vi "Auto 11.vi"(8 "Error In":errorcluster) -> (0 "Error Out":errorcluster)   [LabVIEW 2014]
uses:
  Global Variables/Refnum Names.vi
  <vilib>/Rock Robotics/Network Tables/SD Read Number.vi
  <vilib>/Rock Robotics/Network Tables/SD Read Boolean.vi
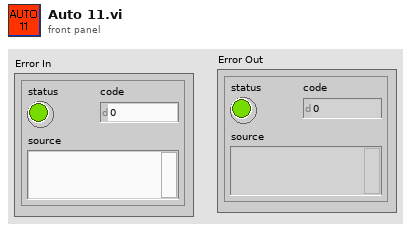
[diagram p1: front panel]
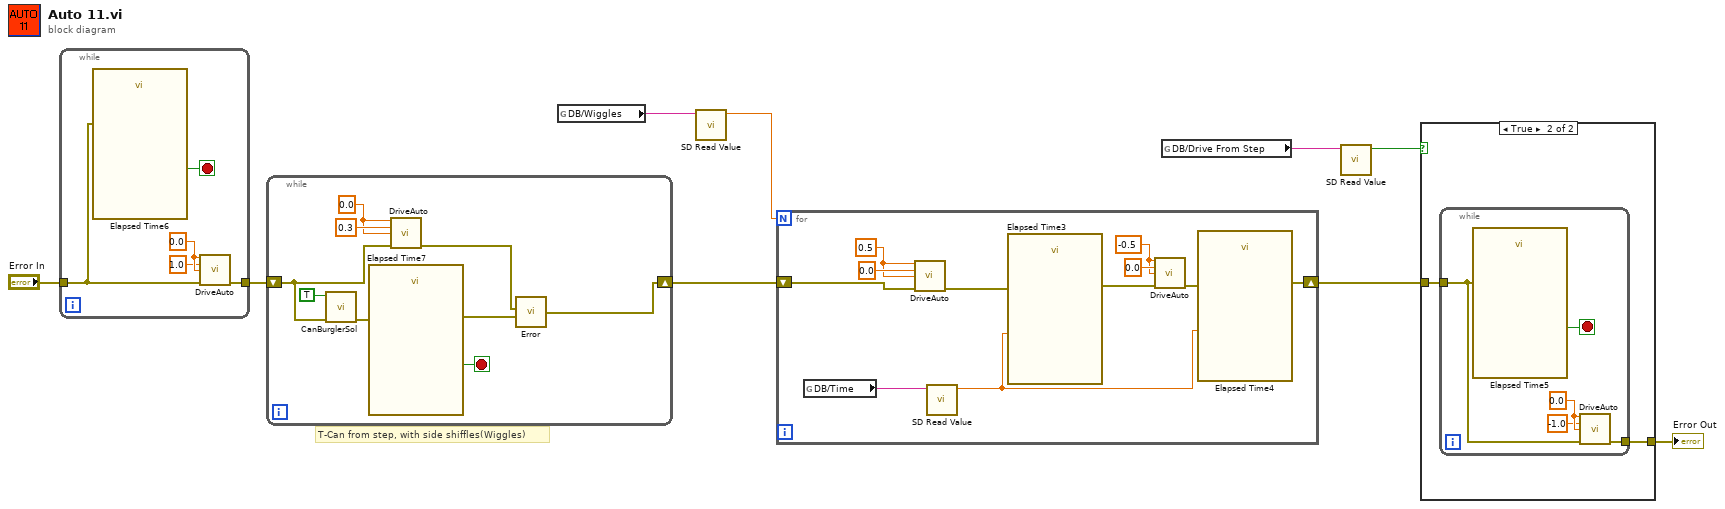
[diagram p0: block diagram]
diagram:
  # "T-Can from step, with side shiffles(Wiggles)"
  n1 = while {
    tunnel: [w14] -> w6
    tunnel: "Error In" -> [w11]
    stop <- w12 stop-if-true
    w13 = 0.0 ("Arm Value")
    n2 = call "Elapsed Time6"("error in (no error)"=w11) -> ("Time has Elapsed"=w12:bool)  [unwired: 11 in, 7 out]
    n3 = call "DriveAuto.vi"("X In"=w13, "Y In"=1.0 ("X In"), "R In"=w13, "Error In"=w11) -> ("Error Out"=w14:errorcluster)  [unwired: 11 in]
  }
  n4 = while {
    shift-right: [w16] -> w4
    shift-left: w6 -> [w19]
    stop <- w22 stop-if-true
    w20 = 0.0 ("Arm Value")
    n5 = call "CanBurglerSol.vi"("Error In"=w19, "Grabber Open/Close"=TRUE) -> ("Error Out"=w23:errorcluster)  [unwired: 9 in]
    n6 = call "Elapsed Time7"("error in (no error)"=w23) -> ("Time has Elapsed"=w22:bool, "error out"=w17:errorcluster)  [unwired: 11 in, 6 out]
    n7 = call "DriveAuto.vi"("X In"=w20, "Y In"=0.3 ("X In"), "R In"=w20, "Error In"=w19) -> ("Error Out"=w18:errorcluster)  [unwired: 11 in]
    n8 = call "Error.vi"("error in (no error)"=w17, "error in (no error) 2"=w18) -> ("error out"=w16:errorcluster)  [unwired: 2 in]
  }
  n9 = global read "Refnum Names.vi" "DB/Wiggles"() -> (w3:string)
  n10 = call-poly <vilib>:"SD Read Value.vi"("Name"=w3) -> ("Numeric"=w7:dbl)  [unwired: 8 in, 2 out]
  n11 = for {
    N: w7 -> [_]
    shift-right: [w28] -> w9
    shift-left: w4 -> [w30]
    w26 = -0.5 ("Arm Value")
    w27 = 0.5 ("Arm Value")
    n12 = global read "Refnum Names.vi" "DB/Time"() -> (w24:string)
    n13 = call "DriveAuto.vi"("X In"=w27, "Y In"=0.0 ("X In"), "R In"=w27, "Error In"=w30) -> ("Error Out"=w33:errorcluster)  [unwired: 11 in]
    n14 = call-poly <vilib>:"SD Read Value.vi"("Name"=w24) -> ("Numeric"=w25:dbl)  [unwired: 8 in, 2 out]
    n15 = call "Elapsed Time3"("Time Target (s)"=w25, "error in (no error)"=w33) -> ("error out"=w29:errorcluster)  [unwired: 10 in, 7 out]
    n16 = call "DriveAuto.vi"("X In"=w26, "Y In"=0.0 ("X In"), "R In"=w26, "Error In"=w29) -> ("Error Out"=w32:errorcluster)  [unwired: 11 in]
    n17 = call "Elapsed Time4"("Time Target (s)"=w25, "error in (no error)"=w32) -> ("error out"=w28:errorcluster)  [unwired: 10 in, 7 out]
  }
  n18 = global read "Refnum Names.vi" "DB/Drive From Step"() -> (w2:string)
  n19 = call-poly <vilib>:"SD Read Value.vi"("Name"=w2) -> ("Boolean"=w1:bool)  [unwired: 8 in, 2 out]
  n20 = case shown="True" w1 {
    tunnel: w9 -> [w35 w37]
    tunnel: [w35 w36] -> w8
    frame False {
    }
    frame True {
      n21 = while {
        tunnel: [w42] -> w36
        tunnel: w37 -> [w39]
        stop <- w40 stop-if-true
        w41 = 0.0 ("Arm Value")
        n22 = call "Elapsed Time5"("error in (no error)"=w39) -> ("Time has Elapsed"=w40:bool)  [unwired: 11 in, 7 out]
        n23 = call "DriveAuto.vi"("X In"=w41, "Y In"=-1.0 ("X In"), "R In"=w41, "Error In"=w39) -> ("Error Out"=w42:errorcluster)  [unwired: 11 in]
      }
    }
  }
  "Error Out" <- w8
